vi "WriteSetPoint.vi"(8 "error in (no error)":errorcluster, 9 "Setpoint (C)":dbl=265.0 format="%.2f", 10 "Port Number":u16=2000, 11 "IP Address":string="192.168.12.201") -> (0 "error out":errorcluster, 3 "Output Reading":string="W01")   [LabVIEW 2013, in "ovenCtrl.lvlib"]
uses:
  ovenCtrl.lvlib
panel:
  # "Inputs"
  # "x.200: Na Reservoir\nx.201: Nozzle"
  # "Outputs"
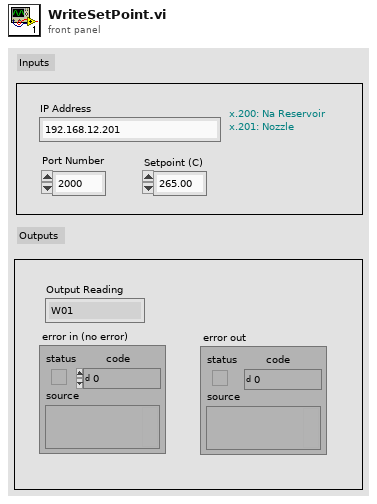
[diagram p1: front panel]
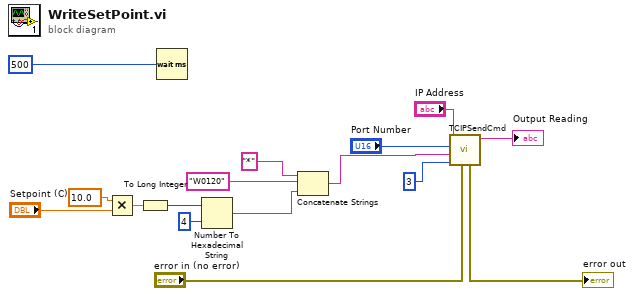
[diagram p0: block diagram]
diagram:
  n1 = Multiply(x=10.0, y="Setpoint (C)") -> (x*y=w13:dbl)
  n2 = To Long Integer(number=w13) -> (32bit integer=w11:i32)
  n3 = Wait (ms)(milliseconds to wait=u32 500) -> ()  [unwired: 1 out]
  n4 = Number To Hexadecimal String(1:i16 4 ("width (-)"), 2:w11) -> (0:w8:string)
  n5 = Concatenate Strings("*" ("string"), "W0120" ("string"), w8) -> (w4:string)
  n6 = call "TCIPSendCmd.vi"("error in (no error)"="error in (no error)", "bytes to read"=3, "Command"=w4, "Port Number"="Port Number", "IP Address"="IP Address") -> ("Output Reading"=→"Output Reading":string, "error out"=→"error out":errorcluster)  [unwired: 5 in]
